vi "习题.vi"() -> ()   [LabVIEW 2023]
panel:
  out "sorted array 2":string[](array[string])
  in  "List 4":string[](array[string])
  in  "List 3":string[](array[string])
  out "sorted array":string[](array[string])
  in  "List 2":string[](array[string])
  in  "List 1":string[](array[string])
  # "习题：\n有两个数组常量，它们都是字符串类型的一维数组，每个数组中都存放了一些小朋友的名字。编写一个 VI 把所有小朋友的名字合并到一个数组中，并且按照字母顺序排序。"
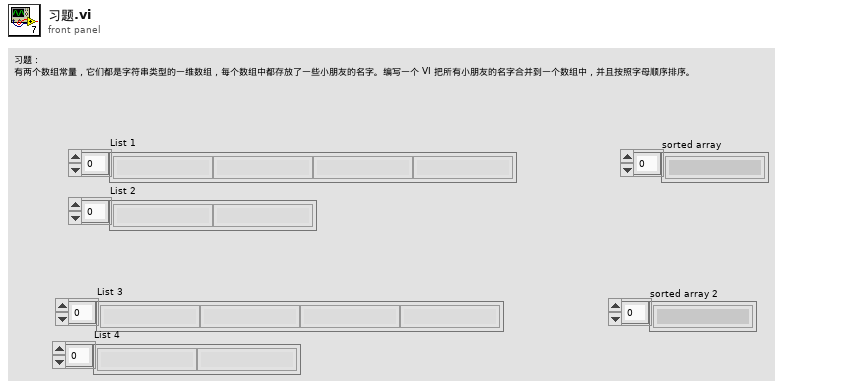
[diagram p1: front panel]
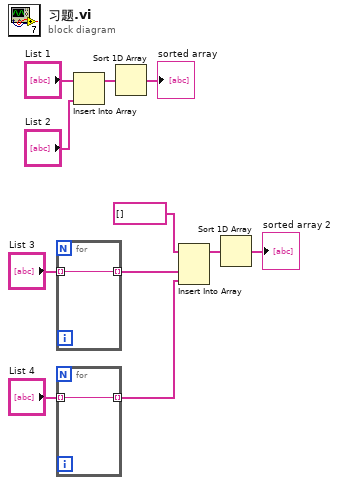
[diagram p0: block diagram]
diagram:
  n1 = for {
    tunnel: "List 3" -> [w12] mode=indexing
    tunnel: [w12] -> w4 mode=indexing
  }
  n2 = for {
    tunnel: "List 4" -> [w13] mode=indexing
    tunnel: [w13] -> w3 mode=indexing
  }
  n3 = Insert Into Array(array="List 1", new element="List 2") -> (w9:string[])  [unwired: 1 in]
  n4 = Sort 1D Array(array=w9) -> (sorted array=→"sorted array":string[])
  n5 = Insert Into Array(array=string[] [], new element #1=w4, new element #2=w3) -> (w2:string[])  [unwired: 1 in]
  n6 = Sort 1D Array(array=w2) -> (sorted array=→"sorted array 2":string[])
